vi "Initialize.vi"(6 "optional":variant, 8 "error in":errorcluster, 11 "Parameter in":refnum<class "Parameter.lvclass">) -> (0 "error out":errorcluster, 3 "Node*":refnum<data-value>)   [LabVIEW 2013, in "Parameter.lvclass"]
doc: "Initializes a node. Makes a data value reference of the node, sets the selfNode, and output the data value reference."
uses:
  Parameter.lvclass
  xCE/xceNode/xceNode.lvclass
  xCE/xceDataNode/xceDataNode.lvclass
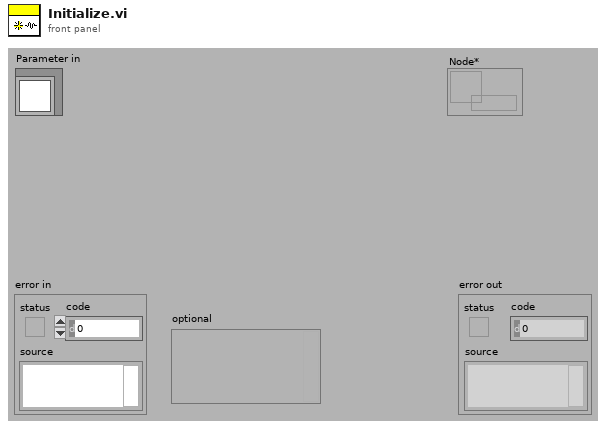
[diagram p1: front panel]
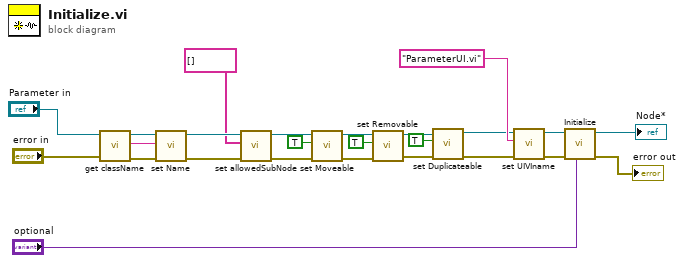
[diagram p0: block diagram]
diagram:
  n1 = call "get className.vi"("error in (no error)"="error in", "xceNode in"="Parameter in") -> ("error out"=w7:errorcluster, "Class name"=w6:string, "xceNode out"=w8:refnum<class "Parameter.lvclass">)  [unwired: 7 in]
  n2 = call "set Name.vi"("error in (no error)"=w7, "Name"=w6, "xceDataNode in"=w8) -> ("error out"=w13:errorcluster, "xceDataNode out"=w12:refnum<class "Parameter.lvclass">)  [unwired: 7 in]
  n3 = call "set allowedSubNode.vi"("error in (no error)"=w13, "Allowed subNode[]"=string[] [], "xceDataNode in"=w12) -> ("error out"=w15:errorcluster, "xceDataNode out"=w14:refnum<class "Parameter.lvclass">)  [unwired: 7 in]
  n4 = call "set Moveable.vi"("error in (no error)"=w15, "Moveable"=TRUE, "xceDataNode in"=w14) -> ("error out"=w18:errorcluster, "xceDataNode out"=w17:refnum<class "Parameter.lvclass">)  [unwired: 7 in]
  n5 = call "set Removable.vi"("error in (no error)"=w18, "Removable"=TRUE, "xceDataNode in"=w17) -> ("error out"=w21:errorcluster, "xceDataNode out"=w20:refnum<class "Parameter.lvclass">)  [unwired: 7 in]
  n6 = call "set Duplicateable.vi"("error in (no error)"=w21, "Duplicateable"=TRUE, "xceDataNode in"=w20) -> ("error out"=w24:errorcluster, "xceDataNode out"=w23:refnum<class "Parameter.lvclass">)  [unwired: 7 in]
  n7 = call "set UIVIname.vi"("error in (no error)"=w24, "UI VI name"="ParameterUI.vi", "xceDataNode in"=w23) -> ("error out"=w2:errorcluster, "xceDataNode out"=w5:refnum<class "Parameter.lvclass">)  [unwired: 7 in]
  n8 = call-parent "Initialize.vi"("optional"="optional", "error in"=w2, "xceDataNode in"=w5) -> ("error out"=→"error out":errorcluster, "Node*"=→"Node*":refnum<data-value>)  [unwired: 7 in]
